vi "Logs.vi"(7 "Action":enum8{"noop", "add", "clear"}(ring), 11 "log":cluster{"time":timestamp, "error":errorcluster}) -> (3 "logs":T1(array[cluster]))   [LabVIEW 2021, in "HttpServer.lvlib"]
uses:
  HttpServer.lvlib
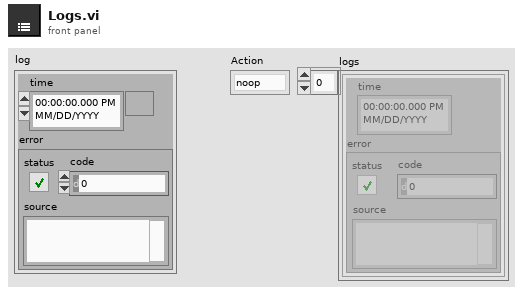
[diagram p1: front panel]
types:
  T1 = cluster{"time":timestamp, "error":errorcluster}[]
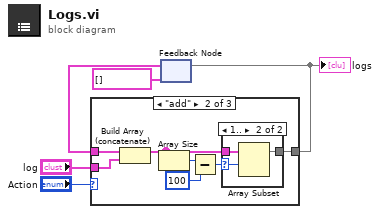
[diagram p0: block diagram]
diagram:
  n1 = feedback #1(T1 []) -> (w2:T1)
  n2 = case shown="\"add\"" "Action" {
    tunnel: "log" -> [_ w12 _]
    tunnel: w2 -> [w6 w13 _]
    tunnel: [w6 w8 _] -> w1
    frame "noop" {
    }
    frame "add" {
      n3 = Build Array (concatenate)(w13, w12) -> (w9:T1)
      n4 = Array Size(array=w9) -> (size(s)=w11:i32)
      n5 = Subtract(x=w11, y=100) -> (x-y=w7:i32)
      n6 = case shown="1.." w7 {
        selector: w7 -> [_ w15]
        tunnel: w9 -> [w14 w17]
        tunnel: [w14 w16] -> w8
        frame ..0 {
        }
        frame 1.. {
          n7 = Array Subset(array=w17, index=w15) -> (w16:T1)  [unwired: 1 in]
        }
      }
    }
    frame "clear" {
    }
  }
  "logs" <- w1
  n8 = feedback-in #1(w1) -> ()
